vi "SwTmr Save Configuration Settings to XML.vi"(8 "error in (no error)":errorcluster, 11 "User Configuration":T1={"Hardware Configuration"={"Physical Channel"="", "Maximum Input"=0.0, "Minimum Input"=0.0, "Sample Rate"=0.0, "Number of Samples"=0}, "Analysis Configuration"={"Statistics"=TRUE}, "New Data Behavior"=enum."Replace", "Time-Voltage transfer function file path (dialog if empty)"=path "", "Cell (V) Error Upper"=0.0, "Cell (V) Error Lower (type \"-\")"=0.0}) -> (0 "error out":errorcluster)   [LabVIEW 2017]
doc: "Saves the user-specified configuration data to an XML file. This is used to remember settings between executions."
uses:
  controls/SwTmr User Specified Data.ctl
  controls/SwTmr HW Configuration.ctl
  controls/SwTmr Analysis Configuration.ctl
  controls/SwTmr New Data Behavior.ctl
  controls/SwTmr Transfer Func File Path.ctl
  <vilib>/Utility/xml.llb/Write to XML File(string).vi
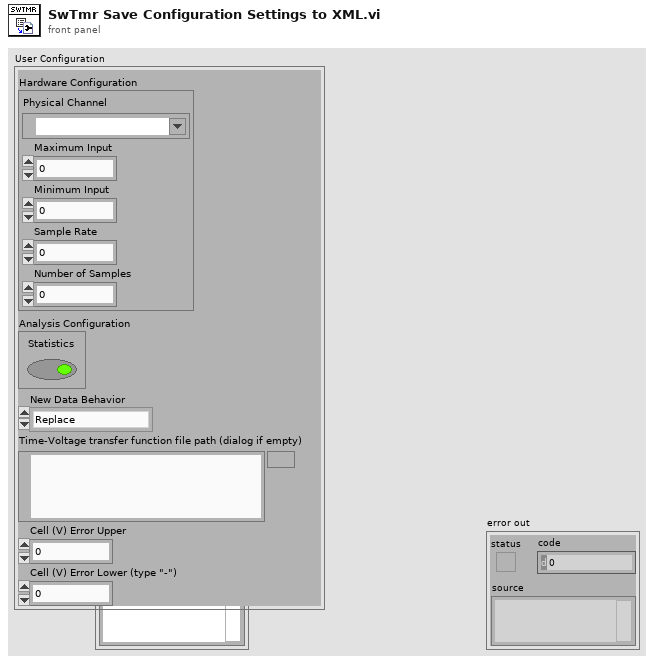
[diagram p1: front panel]
types:
  T1 = typedef "SwTmr User Specified Data.ctl" = cluster{"Hardware Configuration":T2, "Analysis Configuration":T3, "New Data Behavior":T4, "Time-Voltage transfer function file path (dialog if empty)":T5, "Cell (V) Error Upper":dbl, "Cell (V) Error Lower (type \"-\")":dbl}
  T2 = typedef "SwTmr HW Configuration.ctl" = cluster{"Physical Channel":tag, "Maximum Input":dbl, "Minimum Input":dbl, "Sample Rate":dbl, "Number of Samples":i32}
  T3 = typedef "SwTmr Analysis Configuration.ctl" = cluster{"Statistics":bool}
  T4 = typedef "SwTmr New Data Behavior.ctl" = enum16{"Replace", "Overlay", "Append"}
  T5 = typedef "SwTmr Transfer Func File Path.ctl" = path
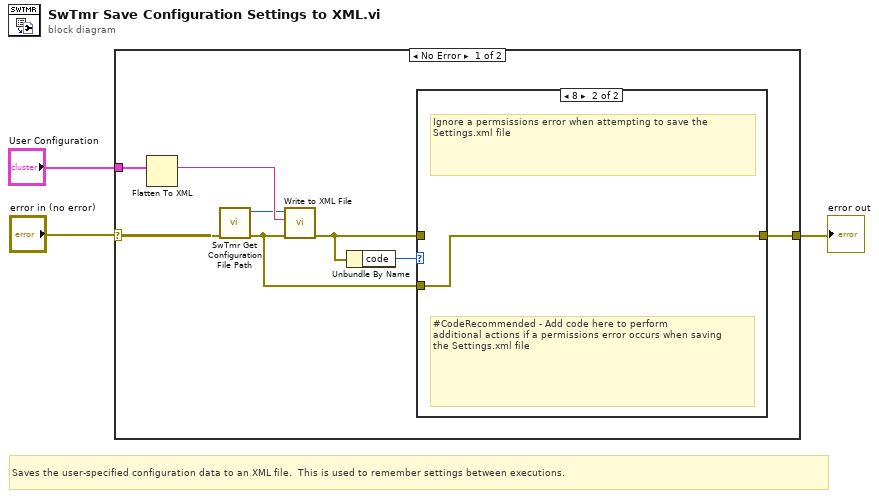
[diagram p0: block diagram]
diagram:
  # "Saves the user-specified configuration data to an XML file.  This is used to remember settings between executions."
  n1 = case shown="No Error" "error in (no error)" {
    selector: "error in (no error)" -> [w8 w14]
    tunnel: [w5 w14] -> w2
    tunnel: "User Configuration" -> [w11 _]
    frame No Error {
      n2 = Flatten To XML(anything=w11) -> (xml string=w10:string)
      n3 = call "SwTmr Get Configuration File Path.vi"("error in (no error)"=w8) -> ("error out"=w4:errorcluster, "XML File Path"=w9:path)  [unwired: 9 in]
      n4 = call-poly <vilib>:"Write to XML File.vi"("error in (no error)"=w4, "XML Input"=w10, "XML File Path"=w9) -> ("error out"=w6:errorcluster)  [unwired: 6 in, 2 out]
      n5 = Unbundle By Name(w6) -> ("code"=w7:i32)
      n6 = case shown="8" w7 {
        tunnel: w6 -> [w12 _]
        tunnel: [w12 w13] -> w5
        tunnel: w4 -> [_ w13]
        frame Default {
        }
        frame 8 {
          # "#CodeRecommended - Add code here to perform\nadditional actions if a permissions error occurs when saving\nthe Settings.xml file"
          # "Ignore a permsissions error when attempting to save the\nSettings.xml file"
        }
      }
    }
    frame Error {
    }
  }
  "error out" <- w2
